vi "NewErriorLoggerFile.vi"(8 "error in (no error)":errorcluster, 9 "ErrorLogPath":path, 10 "Filenumber":u32, 11 "TCP_Client in":refnum<class "TCP_Client.lvclass">) -> (0 "error out":errorcluster, 3 "TCP_Client out":refnum<class "TCP_Client.lvclass">)   [LabVIEW 2023, in "TCP_Client.lvlib" / "TCP_Client.lvclass"]
uses:
  TCP_Client.lvclass
  TCP_Client.lvclass/TCP_Client.ctl
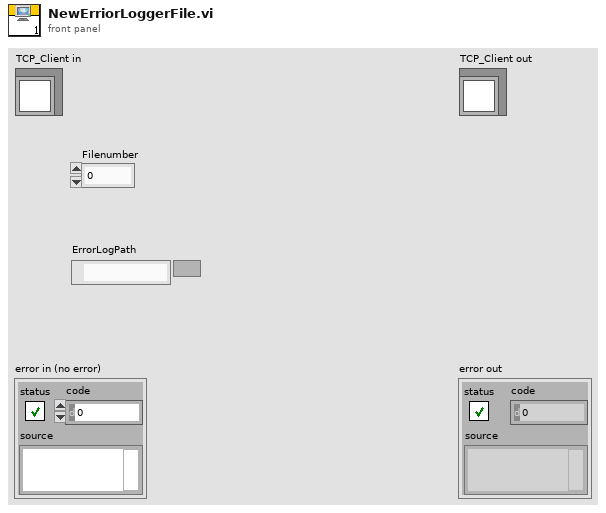
[diagram p1: front panel]
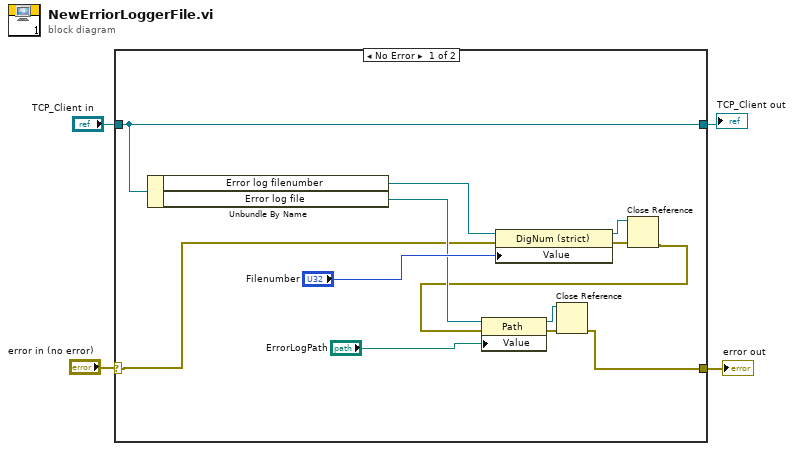
[diagram p0: block diagram]
diagram:
  n1 = case shown="No Error" "error in (no error)" {
    selector: "error in (no error)" -> [w9 w18]
    tunnel: "TCP_Client in" -> [w5 w17]
    tunnel: [w6 w18] -> w2
    tunnel: [w5 w17] -> w1
    frame No Error {
      n2 = Unbundle By Name(w5) -> ("Error log filenumber"=w15:refnum<vi>, "Error log file"=w11:refnum<vi>)
      n3 = property class="DigNum (strict)"(reference=w15, error in=w9, "Value"="Filenumber") -> (reference out=w13:refnum<vi>, error out=w14:errorcluster)
      n4 = Close Reference(reference=w13, error in (no error)=w14) -> (error out=w10:errorcluster)
      n5 = property class="Path"(reference=w11, error in=w10, "Value"="ErrorLogPath") -> (reference out=w7:refnum<vi>, error out=w8:errorcluster)
      n6 = Close Reference(reference=w7, error in (no error)=w8) -> (error out=w6:errorcluster)
    }
    frame Error {
    }
  }
  "error out" <- w2
  "TCP_Client out" <- w1
